vi "Add License to VI Documentation.vi"(6 "Variant in":variant, 7 "Shift Pressed?":bool, 8 "error in (no error)":errorcluster, 10 "QD Combo Box Ref":refnum<vi>, 11 "QD Launch VI Ref":refnum<vi>) -> (0 "error out":errorcluster, 4 "Variant out":variant)   [LabVIEW 2020, in "Add License to VI Documentation.lvlib"]
doc: "This VI adds boiler-plate text to your VI or, if you also hold the Shift key, every VI in your project instance.\n\nDefault Shortcut - [L]"
uses:
  Add License to VI Documentation.lvlib
panel:
  in  "Undo Name":string="Quick Drop Keyboard Shortcut"
  # "Do not change the connector pane of this VI.\n\nSee the block diagram for directions on how to use this template."
  # "Specify the name of the Undo transaction"
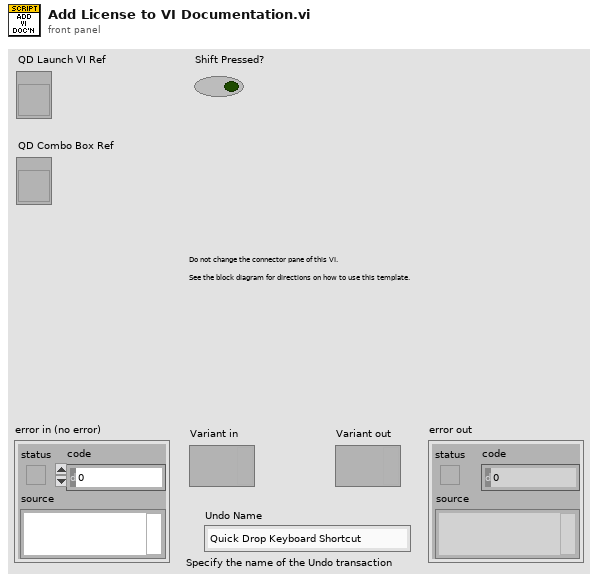
[diagram p1: front panel]
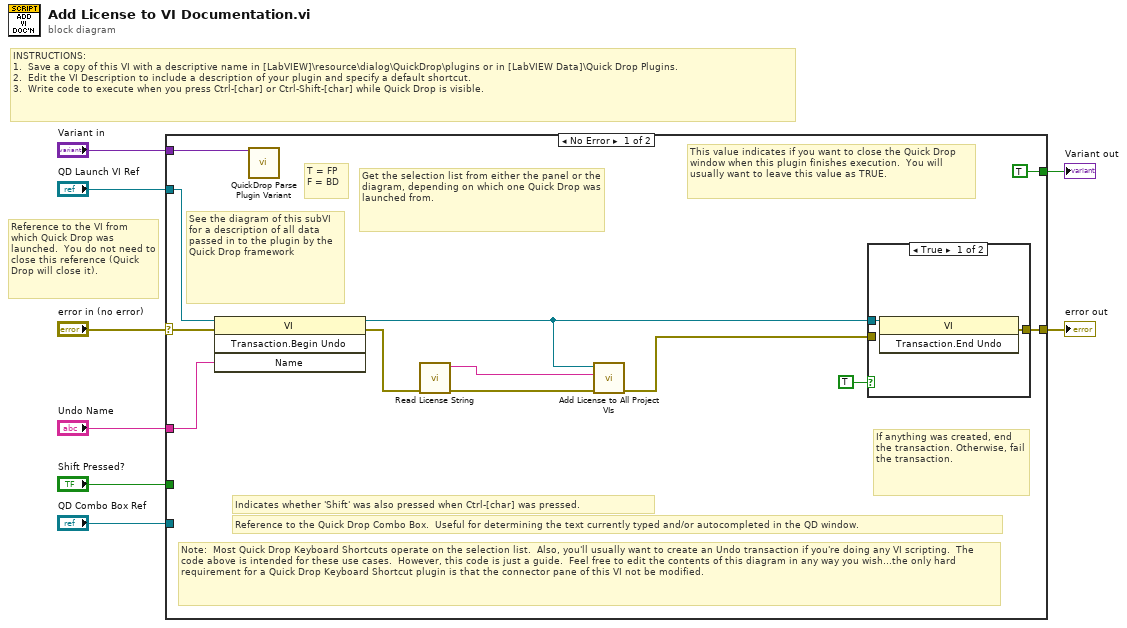
[diagram p0: block diagram]
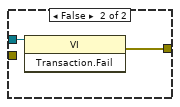
[diagram p2: hidden frame]
diagram:
  # "Reference to the VI from which Quick Drop was launched.  You do not need to close this reference (Quick Drop will close it)."
  # "INSTRUCTIONS:\n1.  Save a copy of this VI with a descriptive name in [LabVIEW]\\resource\\dialog\\QuickDrop\\plugins or in [LabVIEW Data]\\Quick Drop Plugins.\n2.  Edit the VI Description to include a description of your plugin and specify a default shortcut. \n3.  Write code to execute when you press Ctrl-[char] or Ctrl-Shift-[char] while Quick Drop is visible."
  n1 = case shown="No Error" "error in (no error)" {
    selector: "error in (no error)" -> [w19 w25]
    tunnel: [w15 w25] -> w7
    tunnel: "QD Launch VI Ref" -> [w18 _]
    tunnel: "Shift Pressed?" -> [_ _]
    tunnel: "QD Combo Box Ref" -> [_ _]
    tunnel: "Variant in" -> [w20 _]
    tunnel: "Undo Name" -> [w17 _]
    tunnel: [TRUE _] -> w1
    frame No Error {
      # "T = FP\nF = BD"
      # "Note:  Most Quick Drop Keyboard Shortcuts operate on the selection list.  Also, you'll usually want to create an Undo transaction if you're doing any VI scripting.  The code above is intended for these use cases.  However, this code is just a guide.  Feel free to edit the contents of this diagram in any way you wish...the only hard requirement for a Quick Drop Keyboard Shortcut plugin is that the connector pane of this VI not be modified."
      # "Get the selection list from either the panel or the diagram, depending on which one Quick Drop was launched from."
      # "If anything was created, end the transaction. Otherwise, fail the transaction."
      # "This value indicates if you want to close the Quick Drop window when this plugin finishes execution.  You will usually want to leave this value as TRUE."
      # "See the diagram of this subVI for a description of all data passed in to the plugin by the Quick Drop framework"
      # "Reference to the Quick Drop Combo Box.  Useful for determining the text currently typed and/or autocompleted in the QD window."
      # "Indicates whether 'Shift' was also pressed when Ctrl-[char] was pressed."
      n2 = invoke class="VI" method="Transaction.Begin Undo"(reference=w18, error in=w19, "Name"=w17) -> (reference out=w13:refnum<vi>, error out=w10:errorcluster)  [unwired: 1 in, 2 out]
      n3 = call <vilib>:"QuickDrop Parse Plugin Variant.vi"("QDKS Variant in"=w20) -> ()  [unwired: 12 in, 3 out]
      n4 = call "Read License String.vi"("error in (no error)"=w10) -> ("error out"=w9:errorcluster, "License String"=w11:string)  [unwired: 9 in]
      n5 = call "Add License to All Project VIs.vi"("error in (no error)"=w9, "License Text to Add"=w11, "VI in"=w13) -> ("error out"=w12:errorcluster)  [unwired: 8 in]
      n6 = case shown="True" TRUE {
        tunnel: w13 -> [w21 w23]
        tunnel: [w22 w24] -> w15
        tunnel: w12 -> [_ _]
        frame True {
          n7 = invoke class="VI" method="Transaction.End Undo"(reference=w21) -> (error out=w22:errorcluster)  [unwired: 2 in, 2 out]
        }
        frame False {
          n8 = invoke class="VI" method="Transaction.Fail"(reference=w23) -> (error out=w24:errorcluster)  [unwired: 2 in, 2 out]
        }
      }
    }
    frame Error {
    }
  }
  "error out" <- w7
  "Variant out" <- w1
